vi "Delete_Sheet_In_Excel 2010.vi"(8 "error in (no error)":errorcluster, 10 "Master Sheet Name":string="Sheet1", 11 "Excel Path":path=path "C:/Temp/Test.xlsx") -> (0 "error out":errorcluster)   [LabVIEW 2015]
panel:
  in  "Excel._Worksheet":refnum<k7>
  in  "Excel._Application":refnum<k7>
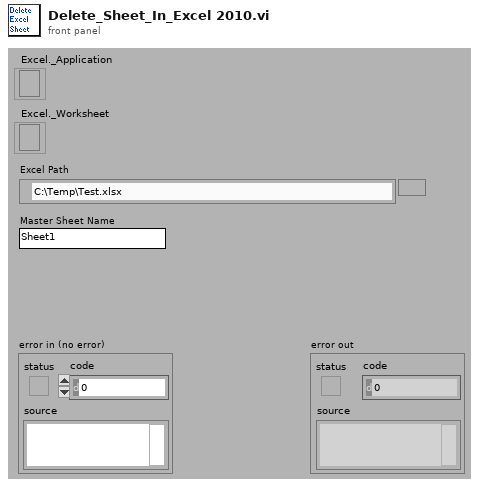
[diagram p1: front panel]
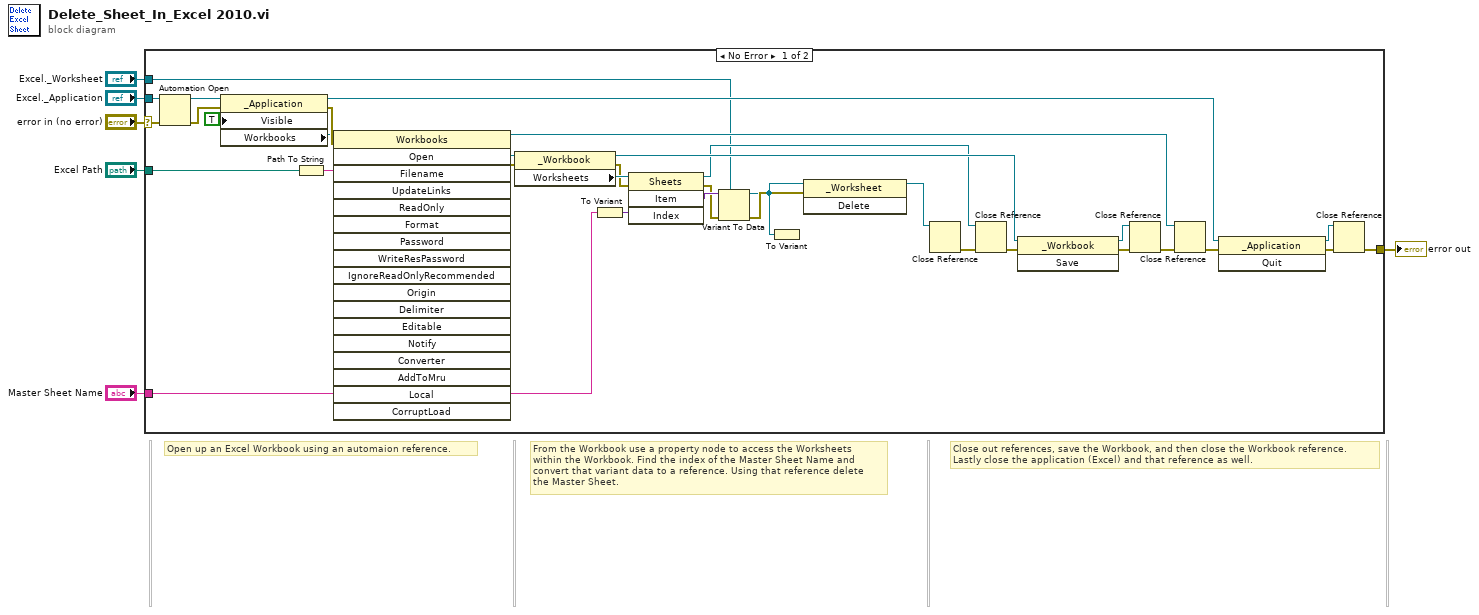
[diagram p0: block diagram]
diagram:
  # "Close out references, save the Workbook, and then close the Workbook reference.\nLastly close the application (Excel) and that reference as well."
  # "From the Workbook use a property node to access the Worksheets \nwithin the Workbook. Find the index of the Master Sheet Name and \nconvert that variant data to a reference. Using that reference delete\nthe Master Sheet."
  # "Open up an Excel Workbook using an automaion reference."
  n1 = case shown="No Error" "error in (no error)" {
    selector: "error in (no error)" -> [w23 w41]
    tunnel: "Excel._Worksheet" -> [w9 _]
    tunnel: [w34 w41] -> w5
    tunnel: "Excel._Application" -> [w30 _]
    tunnel: "Excel Path" -> [w28 _]
    tunnel: "Master Sheet Name" -> [w7 _]
    frame No Error {
      n2 = Automation Open(error in (no error)=w23, Automation Refnum=w30) -> (Automation Refnum=w31:refnum<k7>, error out=w40:errorcluster)  [unwired: 2 out]
      n3 = property class="_Application"(reference=w31, error in=w40, "Visible"=TRUE) -> (reference out=w15:refnum<k7>, error out=w21:errorcluster, "Workbooks"=w20:refnum<k7>)
      n4 = Path To String(path=w28) -> (string=w27:string)
      n5 = invoke class="Workbooks" method="Open"(reference=w20, error in=w21, "Filename"=w27) -> (reference out=w26:refnum<k7>, error out=w24:errorcluster, "Open"=w25:refnum<k7>)  [unwired: 15 in, 15 out]
      n6 = property class="_Workbook"(reference=w25, error in=w24) -> (reference out=w11:refnum<k7>, error out=w18:errorcluster, "Worksheets"=w19:refnum<k7>)
      n7 = To Variant(anything=w7) -> (Variant=w8:variant)
      n8 = invoke class="Sheets" method="Item"(reference=w19, error in=w18, "Index"=w8) -> (reference out=w10:refnum<k7>, error out=w16:errorcluster, "Item"=w17:variant)  [unwired: 1 in, 1 out]
      n9 = Variant To Data(error in=w16, type=w9, Variant=w17) -> (data=w13:refnum<k7>, error out=w14:errorcluster)
      n10 = To Variant(anything=w13) -> ()  [unwired: 1 out]
      n11 = invoke class="_Worksheet" method="Delete"(reference=w13, error in=w14) -> (reference out=w12:refnum<k7>)  [unwired: 1 in, 2 out]
      n12 = Close Reference(reference=w12) -> (error out=w22:errorcluster)  [unwired: 1 in]
      n13 = Close Reference(reference=w10, error in (no error)=w22) -> (error out=w29:errorcluster)
      n14 = invoke class="_Workbook" method="Save"(reference=w11, error in=w29) -> (reference out=w37:refnum<k7>, error out=w38:errorcluster)  [unwired: 1 in, 1 out]
      n15 = Close Reference(reference=w37, error in (no error)=w38) -> (error out=w36:errorcluster)
      n16 = Close Reference(reference=w26, error in (no error)=w36) -> (error out=w33:errorcluster)
      n17 = invoke class="_Application" method="Quit"(reference=w15, error in=w33) -> (reference out=w32:refnum<k7>, error out=w35:errorcluster)  [unwired: 1 in, 1 out]
      n18 = Close Reference(reference=w32, error in (no error)=w35) -> (error out=w34:errorcluster)
    }
    frame Error {
    }
  }
  "error out" <- w5
